vi "UE_Send.vi"(8 "error in (no error)":errorcluster, 9 "Payload":string, 10 "Cmd":string, 11 "UI_Actor in":refnum<class "UI_Actor.lvclass">) -> (0 "error out":errorcluster, 3 "UI_Actor out":refnum<class "UI_Actor.lvclass">)   [LabVIEW 2020, in "UI_Actor.lvlib" / "UI_Actor.lvclass"]
uses:
  UI_Actor.lvclass
  ctl_UE_Msg.ctl
  UI_Actor.lvclass/UI_Actor.ctl
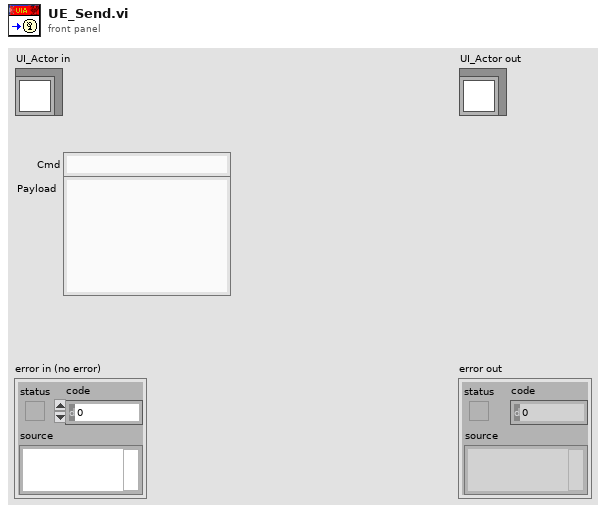
[diagram p1: front panel]
types:
  T1 = typedef "UI_Actor.lvlib/UI_Actor.lvclass/ctl_UE_Msg.ctl" = cluster{"Cmd":string, "Payload":string}
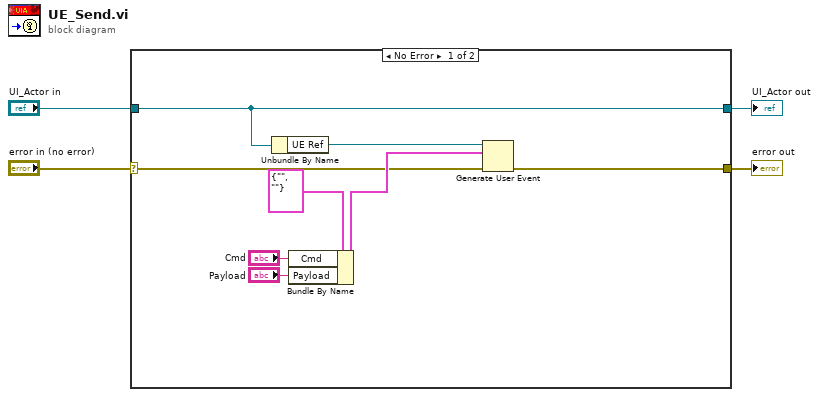
[diagram p0: block diagram]
diagram:
  n1 = case shown="No Error" "error in (no error)" {
    selector: "error in (no error)" -> [w8 w14]
    tunnel: [w7 w14] -> w3
    tunnel: [w12 w13] -> w1
    tunnel: "UI_Actor in" -> [w12 w13]
    frame No Error {
      n2 = Unbundle By Name(w12) -> ("UE Ref"=w11:refnum<user-event>)
      n3 = Bundle By Name(cluster=T1 {"Cmd"="", "Payload"=""} ("event data"), "Cmd"="Cmd", "Payload"="Payload") -> (w9:T1)
      n4 = Generate User Event(user event=w11, event data cluster=w9, error in=w8) -> (error out=w7:errorcluster)  [unwired: 1 in, 1 out]
    }
    frame Error {
    }
  }
  "error out" <- w3
  "UI_Actor out" <- w1
